vi "Extract Multiplier.vi"(11 "Message":u8[](array[numeric]) format="%.0x") -> (0 "State 1":enum16{"OFF", "AC", "DC", "AC+DC"}(ring), 1 "Range (0..6)":i32, 2 "Function (0..15)":T1, 3 "Multiplier":dbl, 4 "State 2":enum16{"OFF", "Auto", "Manual", "Undefined"}(ring))   [LabVIEW 2015, in "VC940.lvlib"]
uses:
  VC940.lvlib
  Controls/Function.ctl
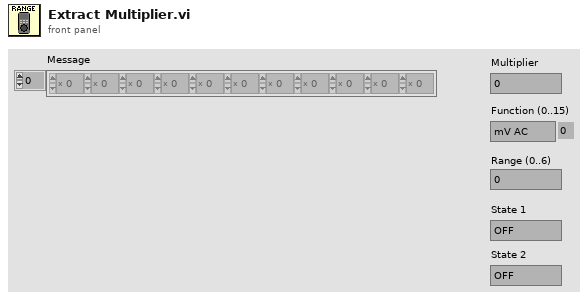
[diagram p1: front panel]
types:
  T1 = typedef "VC940.lvlib/Function.ctl" = enum8{"mV AC", "V DC", "V AC", "mV DC", "Ohm", "nF", "°C", "µA", "mA", "A", "Ohm Fm", "V Diode", "Hz", "°F", "W", "%4-20mA"}
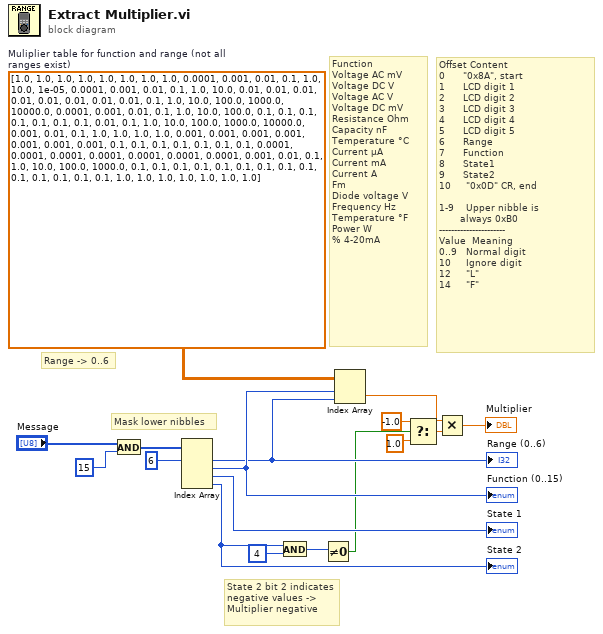
[diagram p0: block diagram]
diagram:
  w11 = dbl[][] [[1.0, 1.0, 1.0, 1.0, 1.0, 1.0, 1.0], [1.0, 0.0001, 0.001, 0.01, 0.1, 1.0, 10.0], [1e-05, 0.0001, 0.001, 0.01, 0.1, 1.0, 10.0], [0.01, 0.01, 0.01, 0.01, 0.01, 0.01, 0.01], [0.01, 0.1, 1.0, 10.0, 100.0, 1000.0, 10000.0], [0.0001, 0.001, 0.01, 0.1, 1.0, 10.0, 100.0], [0.1, 0.1, 0.1, 0.1, 0.1, 0.1, 0.1], [0.01, 0.1, 1.0, 10.0, 100.0, 1000.0, 10000.0], [0.001, 0.01, 0.1, 1.0, 1.0, 1.0, 1.0], [0.001, 0.001, 0.001, 0.001, 0.001, 0.001, 0.001], [0.1, 0.1, 0.1, 0.1, 0.1, 0.1, 0.1], [0.0001, 0.0001, 0.0001, 0.0001, 0.0001, 0.0001, 0.0001], [0.001, 0.01, 0.1, 1.0, 10.0, 100.0, 1000.0], [0.1, 0.1, 0.1, 0.1, 0.1, 0.1, 0.1], [0.1, 0.1, 0.1, 0.1, 0.1, 0.1, 0.1], [1.0, 1.0, 1.0, 1.0, 1.0, 1.0, 1.0]]  # Muliplier table for function and range (not all ranges exist)
  # "Range -> 0..6"
  # "Function\nVoltage AC mV\nVoltage DC V\nVoltage AC V\nVoltage DC mV\nResistance Ohm\nCapacity nF\nTemperature °C\nCurrent µA\nCurrent mA\nCurrent A\nFm\nDiode voltage V\nFrequency Hz\nTemperature °F\nPower W\n% 4-20mA"
  # "Offset Content\n0      \"0x8A\", start\n1      LCD digit 1\n2      LCD digit 2\n3      LCD digit 3\n4      LCD digit 4\n5      LCD digit 5\n6      Range\n7      Function\n8      State1\n9      State2\n10     \"0x0D\" CR, end\n\n1-9    Upper nibble is\n       always 0xB0\n----------------------\nValue  Meaning\n0..9   Normal digit\n10     Ignore digit\n12     \"L\"\n14     \"F\""
  # "Mask lower nibbles"
  # "State 2 bit 2 indicates\nnegative values ->\nMultiplier negative"
  n1 = And(x="Message", y=u8 15) -> (x .and. y?=w15:u8[])
  n2 = Index Array(array=w15, index #1=6 ("index")) -> (element #1=w12:u8, element #2=w13:u8, element #3=→"State 1":u8, element #4=w8:u8)  [unwired: 3 in]
  "Range (0..6)" <- w12
  "Function (0..15)" <- w13
  "State 2" <- w8
  n3 = And(x=w8, y=u8 4) -> (x .and. y?=w10:u8)
  n4 = Not Equal To 0?(x=w10) -> (x != 0?=w3:bool)
  n5 = Index Array(array=w11, index (row)=w13, index (col)=w12) -> (element=w4:dbl)
  n6 = Select(t=-1.0, s=w3, f=1.0 ("t")) -> (s? t:f=w5:dbl)
  n7 = Multiply(x=w4, y=w5) -> (x*y=→"Multiplier":dbl)
